vi "Begin.vi"(11 "Image Size":T1=enum."160x120") -> (0 "error out":errorcluster)   [LabVIEW 2012]
doc: "Called before other user functions, this VI is expected to open initial I/O refnums, load in file data, and do all program initialization. Notice that the <B>error out</B> terminal is simply used for data flow. Wiring it to other structures or subVIs ensures that this VI runs first."
uses:
  <vilib>/Rock Robotics/WPI/Camera/WPI_CameraImageSize.ctl
  <vilib>/Rock Robotics/WPI/Joystick/WPI_JoystickDeviceEnum.ctl
  <vilib>/Rock Robotics/WPI/Camera/WPI_CameraWhite Balance Values.ctl
  <vilib>/Rock Robotics/WPI/Camera/WPI_CameraExposure Values.ctl
  <vilib>/Rock Robotics/WPI/Camera/WPI_CameraFrameRate.ctl
  <vilib>/Rock Robotics/SystemInterfaces/DIO/FPGA_DIOPWMChannel.ctl
  <vilib>/Rock Robotics/SystemInterfaces/Typedef/FPGA_TypedefDigitalModule.ctl
  <vilib>/Rock Robotics/SystemInterfaces/DIO/FPGA_DIOChannel.ctl
  <vilib>/Rock Robotics/SystemInterfaces/DIO/FPGA_DIORelayChannel.ctl
  <vilib>/Rock Robotics/SystemInterfaces/Typedef/FPGA_TypedefSolenoidModule.ctl
  <vilib>/Rock Robotics/WPI/Solenoid/WPI_SolenoidChannel.ctl
  <vilib>/Rock Robotics/WPI/Encoder/WPI_EncoderType.ctl
  <vilib>/Rock Robotics/WPI/RobotDrive/WPI_RobotDriveOpen4MotorWithVictor.vi
  <vilib>/Rock Robotics/WPI/Solenoid/WPI_SolenoidOpenSingle.vi
  <vilib>/Rock Robotics/WPI/Counter/WPI_CounterDigitalInputToDigitalSource.vi
  <vilib>/Rock Robotics/WPI/Compressor/WPI_CompressorGetSetRefNum.vi
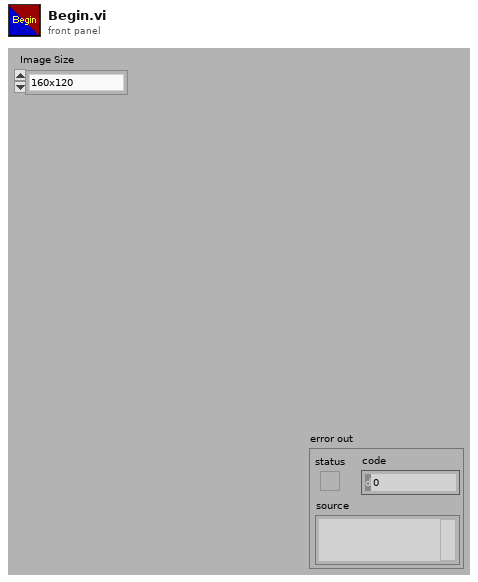
[diagram p1: front panel]
types:
  T1 = typedef "WPI_CameraImageSize.ctl" = enum16{"640x480", "320x240", "160x120"}
  T2 = typedef "WPI_EncoderType.ctl" = enum16{"1x", "2x", "4x"}
  T3 = typedef "FPGA_DIOChannel.ctl" = enum8{"DIO 1", "DIO 2", "DIO 3", "DIO 4", "DIO 5", "DIO 6", "DIO 7", "DIO 8", "DIO 9", "DIO 10", "DIO 11", "DIO 12", "DIO 13", "DIO 14", "Invalid"}
  T4 = typedef "FPGA_TypedefDigitalModule.ctl" = enum16{"Digital Module 1", "Digital Module 2"}
  T5 = typedef "WPI_SolenoidChannel.ctl" = enum8{"Solenoid 1", "Solenoid 2", "Solenoid 3", "Solenoid 4", "Solenoid 5", "Solenoid 6", "Solenoid 7", "Solenoid 8", "Invalid"}
  T6 = typedef "FPGA_TypedefSolenoidModule.ctl" = enum16{"Solenoid Module 1", "Solenoid Module 2"}
  T7 = typedef "FPGA_DIORelayChannel.ctl" = enum8{"Relay 1", "Relay 2", "Relay 3", "Relay 4", "Relay 5", "Relay 6", "Relay 7", "Relay 8", "Invalid"}
  T8 = typedef "WPI_JoystickDeviceEnum.ctl" = enum16{"USB 1", "USB 2", "USB 3", "USB 4", "Kinect 1", "Kinect 2"}
  T9 = typedef "FPGA_DIOPWMChannel.ctl" = enum8{"PWM 1", "PWM 2", "PWM 3", "PWM 4", "PWM 5", "PWM 6", "PWM 7", "PWM 8", "PWM 9", "PWM 10", "Invalid"}
  T10 = typedef "WPI_CameraFrameRate.ctl" = u32
  T11 = typedef "WPI_CameraExposure Values.ctl" = enum16{"Auto", "Flicker-free 50 Hz", "Flicker-free 60 Hz", "Hold current"}
  T12 = typedef "WPI_CameraWhite Balance Values.ctl" = enum16{"Auto", "Fixed indoor", "Fixed outdoor 1", "Fixed outdoor 2", "Fixed fluorescent 1", "Fixed fluorescent 2", "Hold current"}
  T13 = typedef "WPI_DigitalInputDevRef.ctl" = cluster{"DevStatus":errorcluster, "DIO Channel":T3, "Digital Module":T4}
  T14 = typedef "FPGA_CounterEncoderSourceConvertionLVSourceType.ctl" = cluster{"DevStatus":errorcluster, "AnalogTriggerMode?":bool, "DigitalMode":cluster{"Digital Module":T4, "DIO Channel":T15}, "AnalogTriggerMode":cluster{"AnalogTriggerIndex":T16, "OutputType":T17}}
  T15 = typedef "FPGA_DIODigitalSourceChannel.ctl" = enum8{"DIO 1", "DIO 2", "DIO 3", "DIO 4", "DIO 5", "DIO 6", "DIO 7", "DIO 8", "DIO 9", "DIO 10", "DIO 11", "DIO 12", "DIO 13", "DIO 14", "Disabled"}
  T16 = typedef "FPGA_AnalogTriggerIndex.ctl" = enum8{"Trig 0", "Trig 1", "Trig 2", "Trig 3", "Trig 4", "Trig 5", "Trig 6", "Trig 7", "Invalid"}
  T17 = typedef "FPGA_AnalogTriggerOutType.ctl" = enum16{"InWindow", "TriggerState", "Rising", "Falling"}
  T18 = typedef "WPI_EncoderDevRef.ctl" = cluster{"DevStatus":errorcluster, "EncoderIndex":T19, "CounterIndex":T20, "DistancePerCount":dbl, "Decoding Type":T2}
  T19 = typedef "FPGA_EncoderIdx.ctl" = enum8{"Enc 0", "Enc 1", "Enc 2", "Enc 3", "Invalid"}
  T20 = typedef "FPGA_CounterCtrSystemIndex.ctl" = enum8{"Ctr 0", "Ctr 1", "Ctr 2", "Ctr 3", "Ctr 4", "Ctr 5", "Ctr 6", "Ctr 7", "Invalid"}
  T21 = typedef "WPI_CameraDevRef.ctl" = cluster{"Camera Address":string, "CameraStatus":errorcluster, "Acquire Image Notifier":refnum<notifier>}
  T22 = typedef "WPI_RobotDriveDevRef.ctl" = cluster{"DevStatus":errorcluster, "Motors[]":T23[], "Square Inputs":bool, "Max Output":dbl, "Isochronous":bool}
  T23 = typedef "WPI_MotorControlDeviceRef.ctl" = cluster{"DeviceStatus":errorcluster, "Type":enum16{"PWM", "CAN"}, "PWM":cluster{"Digital Module":T4, "PWM Channel":T9, "DeadBand":T24}, "CAN":cluster{"Device Number":u8, "Control Mode":T25, "Semaphore":T26, "Max Vout":dbl}, "Invert":bool, "TransformRef":T27, "InvTransformRef":T27}
  T24 = typedef "WPI_PWMDeadband.ctl" = cluster{"Name":string, "maxPositivePwm":i32, "minPositivePwm":i32, "centerPwm":i32, "maxNegativePwm":i32, "minNegativePwm":i32, "angularRange":u16}
  T25 = typedef "WPI_CANJaguar_ControlMode.ctl" = enum8{"Percent VBus", "Current", "Speed", "Position", "Voltage"}
  T26 = typedef "Semaphore RefNum" = refnum<k1>
  T27 = typedef "WPI_PWMTransform_ConPane.ctl" = refnum<vi>
  T28 = typedef "WPI_SolenoidDevRef.ctl" = cluster{"DevStatus":errorcluster, "Solenoid Module":T6, "Forward Solenoid Channel":T5, "Reverse Solenoid Channel":T5}
  T29 = typedef "WPI_JoystickDevRef.ctl" = cluster{"Device":T8}
  T30 = typedef "WPI_CompressorDevRef.ctl" = cluster{"DevStatus":errorcluster, "DigitalInputDevRef":T13, "RelayDevRef":T31}
  T31 = typedef "WPI_RelayDevRef.ctl" = cluster{"DevStatus":errorcluster, "Relay Channel":T7, "Digital Module":T4, "Relay Direction":T32}
  T32 = typedef "WPI_RelayDirection.ctl" = enum16{"Both directions", "Forward only", "Reverse only"}
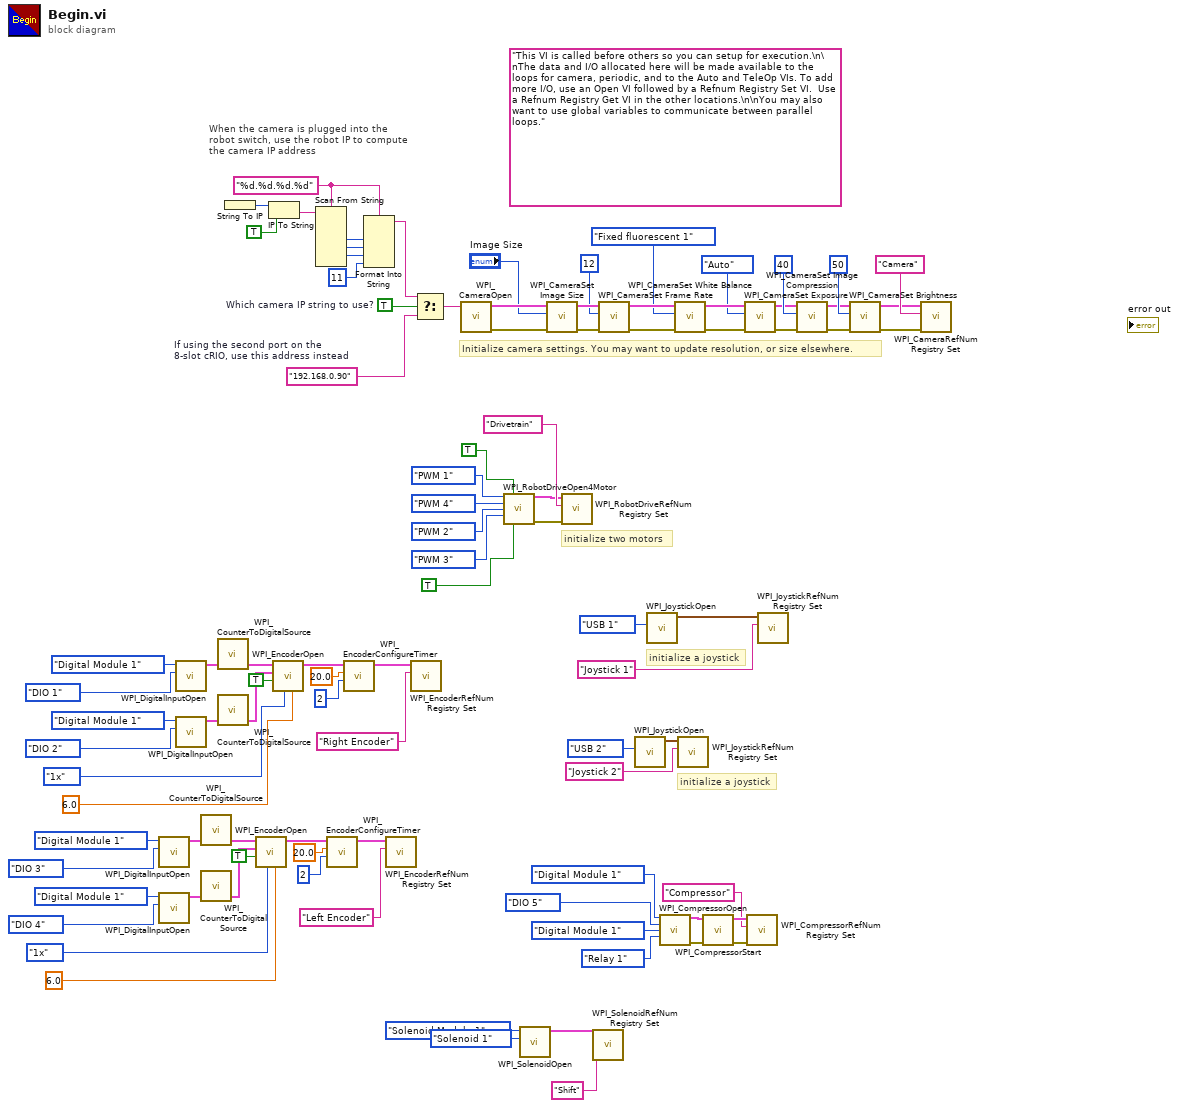
[diagram p0: block diagram]
diagram:
  w57 = TRUE  # Which camera IP string to use?
  w61 = "%d.%d.%d.%d" ("format string")
  (unwired) "This VI is called before others so you can setup for execution.\n\nThe data and I/O allocated here will be made available to the loops for camera, periodic, and to the Auto and TeleOp VIs. To add more I/O, use an Open VI followed by a Refnum Registry Set VI.  Use a Refnum Registry Get VI in the other locations.\n\nYou may also want to use global variables to communicate between parallel loops."
  w58 = "192.168.0.90"  # If using the second port on the 8-slot cRIO, use this address instead
  # "initialize a joystick"
  # "When the camera is plugged into the\nrobot switch, use the robot IP to compute\nthe camera IP address"
  # "initialize a joystick"
  # "initialize two motors"
  # "Initialize camera settings. You may want to update resolution, or size elsewhere."
  n1 = call <vilib>:"WPI_DigitalInputOpen.vi"("DIO Channel"=FPGA_DIOChannel."DIO 3", "Digital Module (Module 1)"=FPGA_TypedefDigitalModule."Digital Module 1") -> ("DigitalInputDevRef"=w21:T13)  [unwired: 8 in, 1 out]
  n2 = call <vilib>:"WPI_DigitalInputOpen.vi"("DIO Channel"=FPGA_DIOChannel."DIO 4", "Digital Module (Module 1)"=FPGA_TypedefDigitalModule."Digital Module 1") -> ("DigitalInputDevRef"=w22:T13)  [unwired: 8 in, 1 out]
  n3 = call <vilib>:"WPI_DigitalInputOpen.vi"("DIO Channel"=FPGA_DIOChannel."DIO 1", "Digital Module (Module 1)"=FPGA_TypedefDigitalModule."Digital Module 1") -> ("DigitalInputDevRef"=w28:T13)  [unwired: 8 in, 1 out]
  n4 = call <vilib>:"WPI_DigitalInputOpen.vi"("DIO Channel"=FPGA_DIOChannel."DIO 2", "Digital Module (Module 1)"=FPGA_TypedefDigitalModule."Digital Module 1") -> ("DigitalInputDevRef"=w30:T13)  [unwired: 8 in, 1 out]
  n5 = call-poly <vilib>:"WPI_CounterToDigitalSource.vi"("DigitalInputDevRef"=w21) -> ("Digital Source"=w16:T14)  [unwired: 6 in]
  n6 = call-poly <vilib>:"WPI_CounterToDigitalSource.vi"("DigitalInputDevRef"=w22) -> ("Digital Source"=w15:T14)  [unwired: 6 in]
  n7 = call-poly <vilib>:"WPI_CounterToDigitalSource.vi"("DigitalInputDevRef"=w28) -> ("Digital Source"=w27:T14)  [unwired: 6 in]
  n8 = call-poly <vilib>:"WPI_CounterToDigitalSource.vi"("DigitalInputDevRef"=w30) -> ("Digital Source"=w29:T14)  [unwired: 6 in]
  n9 = String To IP() -> (0:w68:u32)  [unwired: 1 in]
  n10 = call <vilib>:"WPI_EncoderOpen.vi"("DistancePerCount"=6.0, "Decoding Type"=WPI_EncoderType."1x", "Invert Direction (False)"=TRUE, "BSource"=w15, "ASource"=w16) -> ("EncoderDevRef"=w14:T18)  [unwired: 5 in, 1 out]
  n11 = IP To String(1:TRUE ("dot notation? (F)"), 2:w68) -> (0:w66:string)
  n12 = call <vilib>:"WPI_EncoderOpen.vi"("DistancePerCount"=6.0, "Decoding Type"=WPI_EncoderType."1x", "Invert Direction (False)"=TRUE, "BSource"=w29, "ASource"=w27) -> ("EncoderDevRef"=w12:T18)  [unwired: 5 in, 1 out]
  n13 = Scan From String(format string=w61, input string=w66) -> (output 1=w65:i32, output 2=w64:i32, output 3=w63:i32)  [unwired: 7 in, 3 out]
  n14 = call <vilib>:"WPI_EncoderConfigureTimer.vi"("Number Samples to Average"=u8 2, "Minimum Rate"=20.0, "EncoderDevRef"=w14) -> ("EncoderDevRef"=w13:T18)  [unwired: 7 in, 1 out]
  n15 = call <vilib>:"WPI_EncoderConfigureTimer.vi"("Number Samples to Average"=u8 2, "Minimum Rate"=20.0, "EncoderDevRef"=w12) -> ("EncoderDevRef"=w11:T18)  [unwired: 7 in, 1 out]
  n16 = Format Into String(format string=w61, w65, w64, w63, 11 ("Compression")) -> (resulting string=w59:string)  [unwired: 2 in, 1 out]
  n17 = call <vilib>:"WPI_EncoderRefNum Registry Set.vi"("refnum name"="Left Encoder", "EncoderDevRef"=w13) -> ()  [unwired: 8 in, 2 out]
  n18 = call <vilib>:"WPI_EncoderRefNum Registry Set.vi"("refnum name"="Right Encoder", "EncoderDevRef"=w11) -> ()  [unwired: 8 in, 2 out]
  n19 = Select(t=w59, s=w57, f=w58) -> (s? t:f=w60:string)
  n20 = call <vilib>:"WPI_CameraOpen.vi"("Camera Address"=w60) -> ("error out"=w81:errorcluster, "CameraDevRef"=w82:T21)  [unwired: 1 in, 8 out]
  n21 = call-poly <vilib>:"WPI_RobotDriveOpen4Motor.vi"("Rear Left Motor"=FPGA_DIOPWMChannel."PWM 1", "Rear Left Motor Inverted"=TRUE, "Rear Right Motor"=FPGA_DIOPWMChannel."PWM 4" ("Rear Left Motor"), "Front Left Motor"=FPGA_DIOPWMChannel."PWM 2" ("Rear Left Motor"), "Front Right Motor"=FPGA_DIOPWMChannel."PWM 3" ("Rear Left Motor"), "Front Left Motor Inverted"=TRUE) -> ("RobotDriveDevRef"=w56:T22, "error out"=w55:errorcluster)  [unwired: 8 in]
  n22 = call-poly <vilib>:"WPI_SolenoidOpen.vi"("Solenoid Channel"=WPI_SolenoidChannel."Solenoid 1", "Solenoid Module (Module 1)"=FPGA_TypedefSolenoidModule."Solenoid Module 1") -> ("SolenoidDevRef"=w36:T28)  [unwired: 8 in, 1 out]
  n23 = call <vilib>:"WPI_CameraSet Image Size.vi"("error in (no error)"=w81, "Image Size"="Image Size", "CameraDevRef"=w82) -> ("error out"=w80:errorcluster, "CameraDevRef Out"=w83:T21)  [unwired: 7 out]
  n24 = call <vilib>:"WPI_RobotDriveRefNum Registry Set.vi"("error in (no error)"=w55, "refnum name"="Drivetrain", "RobotDriveDevRef"=w56) -> ()  [unwired: 9 out]
  n25 = call <vilib>:"WPI_SolenoidRefNum Registry Set.vi"("refnum name"="Shift", "SolenoidDevRef"=w36) -> ()  [unwired: 8 in, 2 out]
  n26 = call <vilib>:"WPI_CameraSet Frame Rate.vi"("error in (no error)"=w80, "Frame Rate (fps)"=T10 12, "CameraDevRef"=w83) -> ("error out"=w79:errorcluster, "CameraDevRef Out"=w85:T21)  [unwired: 7 out]
  n27 = call <vilib>:"WPI_JoystickOpen.vi"("JoystickDevice"=WPI_JoystickDeviceEnum."USB 2") -> ("JoystickDevRef"=w50:T29)  [unwired: 10 out]
  n28 = call <vilib>:"WPI_JoystickOpen.vi"("JoystickDevice"=WPI_JoystickDeviceEnum."USB 1") -> ("JoystickDevRef"=w91:T29)  [unwired: 10 out]
  n29 = call <vilib>:"WPI_CompressorOpen.vi"("Pressure Switch Digital Module (Module 1)"=FPGA_TypedefDigitalModule."Digital Module 1", "Pressure Switch DIO Channel"=FPGA_DIOChannel."DIO 5", "Relay Digital Module (Module 1)"=FPGA_TypedefDigitalModule."Digital Module 1", "Relay Channel"=FPGA_DIORelayChannel."Relay 1") -> ("CompressorDevRef"=w43:T30, "error out"=w42:errorcluster)  [unwired: 10 in]
  n30 = call <vilib>:"WPI_CameraSet White Balance.vi"("error in (no error)"=w79, "White Balance"=WPI_CameraWhite_Balance_Values."Fixed fluorescent 1", "CameraDevRef"=w85) -> ("error out"=w78:errorcluster, "CameraDevRef Out"=w84:T21)  [unwired: 7 out]
  n31 = call <vilib>:"WPI_JoystickRefNum Registry Set.vi"("refnum name"="Joystick 2", "JoystickDevRef"=w50) -> ()  [unwired: 1 in, 9 out]
  n32 = call <vilib>:"WPI_CompressorStart.vi"("error in (no error)"=w42, "CompressorDevRef"=w43) -> ("error out"=w45:errorcluster, "CompressorDevRef"=w44:T30)  [unwired: 8 in]
  n33 = call <vilib>:"WPI_CameraSet Exposure.vi"("error in (no error)"=w78, "Exposure"=WPI_CameraExposure_Values."Auto", "CameraDevRef"=w84) -> ("error out"=w77:errorcluster, "CameraDevRef Out"=w87:T21)  [unwired: 7 out]
  n34 = call <vilib>:"WPI_CompressorRefNum Registry Set.vi"("error in (no error)"=w45, "refnum name"="Compressor", "CompressorDevRef"=w44) -> ()  [unwired: 7 in, 2 out]
  n35 = call <vilib>:"WPI_JoystickRefNum Registry Set.vi"("refnum name"="Joystick 1", "JoystickDevRef"=w91) -> ()  [unwired: 1 in, 9 out]
  n36 = call <vilib>:"WPI_CameraSet Image Compression.vi"("error in (no error)"=w77, "Compression"=40, "CameraDevRef"=w87) -> ("error out"=w76:errorcluster, "CameraDevRef Out"=w86:T21)  [unwired: 7 out]
  n37 = call <vilib>:"WPI_CameraSet Brightness.vi"("error in (no error)"=w76, "Brightness"=50, "CameraDevRef"=w86) -> ("error out"=w74:errorcluster, "CameraDevRef Out"=w75:T21)  [unwired: 7 out]
  n38 = call <vilib>:"WPI_CameraRefNum Registry Set.vi"("error in (no error)"=w74, "refnum name"="Camera", "CameraDevRef"=w75) -> ()  [unwired: 9 out]
